vi "fgv_Z-projection image refs.vi"(8 "error in (no error)":errorcluster, 9 "GreenMaxZ":T1, 10 "RedMaxZ":T1, 11 "Function":enum16{"Intialize", "Write", "Read", "Clear"}(ring)) -> (0 "error out":errorcluster, 1 "GreenMaxZ":T1, 2 "RedMaxZ":T1)   [LabVIEW 2020]
uses:
  <vilib>/vision/Image Controls.llb/IMAQ Image.ctl
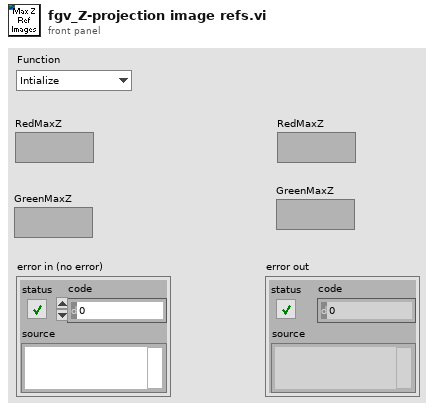
[diagram p1: front panel]
types:
  T1 = typedef "IMAQ Image.ctl" = refnum<image>
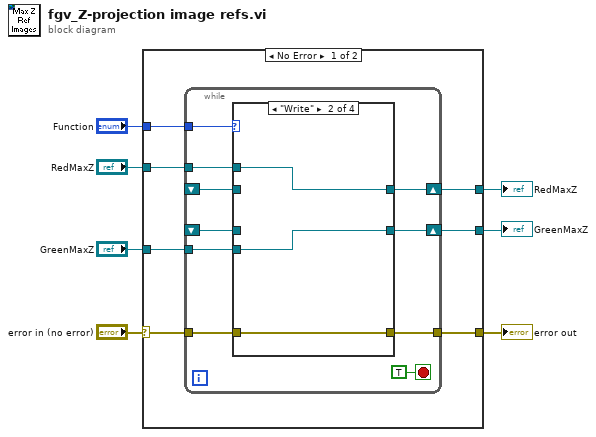
[diagram p0: block diagram]
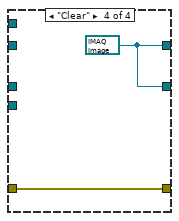
[diagram p4: hidden frame]
diagram:
  n1 = case shown="No Error" "error in (no error)" {
    selector: "error in (no error)" -> [w11 w38]
    tunnel: [w12 w38] -> w6
    tunnel: "Function" -> [w14 _]
    tunnel: "GreenMaxZ" -> [w13 w37]
    tunnel: [w10 w37] -> w1
    tunnel: "RedMaxZ" -> [w9 w36]
    tunnel: [w8 w36] -> w2
    frame No Error {
      n2 = while {
        tunnel: w14 -> [w23]
        tunnel: w13 -> [w22]
        shift-right: [w21] -> w10
        shift-left: _ -> [w20]
        tunnel: [w18] -> w12
        tunnel: w11 -> [w19]
        tunnel: w9 -> [w17]
        shift-right: [w16] -> w8
        shift-left: _ -> [w15]
        stop <- TRUE stop-if-true
        n3 = case shown="\"Write\"" w23 {
          tunnel: [w27 w28 w33 w34] -> w21
          tunnel: w22 -> [_ w28 _ _]
          tunnel: w20 -> [w27 _ w33 _]
          tunnel: [w26 w30 w32 w35] -> w18
          tunnel: w19 -> [w26 w30 w32 w35]
          tunnel: w17 -> [_ w29 _ _]
          tunnel: [w25 w29 w31 w34] -> w16
          tunnel: w15 -> [w25 _ w31 _]
          frame "Intialize", Default {
          }
          frame "Write" {
          }
          frame "Read" {
          }
          frame "Clear" {
            w34 = T1 refnum ("RedMaxZ")
          }
        }
      }
    }
    frame Error {
    }
  }
  "error out" <- w6
  "RedMaxZ" <- w2
  "GreenMaxZ" <- w1
